vi "WriteSettings.vi"(8 "error in (no error)":errorcluster, 10 "Settings":T1, 11 "Controller in":refnum<class "Controller.lvclass">) -> (0 "error out":errorcluster, 3 "Controller out":refnum<class "Controller.lvclass">)   [LabVIEW 2024, in "GUI.lvlib" / "Controller.lvclass"]
uses:
  Controller.lvclass
  Controller.lvclass/Controller.ctl
  <vilib>/drjdpowell/SQLite Library/SQLite.lvlib
  <vilib>/drjdpowell/SQLite Library/SQL Connection/Execute SQL (No results).vi
  <vilib>/drjdpowell/SQLite Library/SQL Connection/Connection.lvclass
  TypeDefs/Settings.ctl
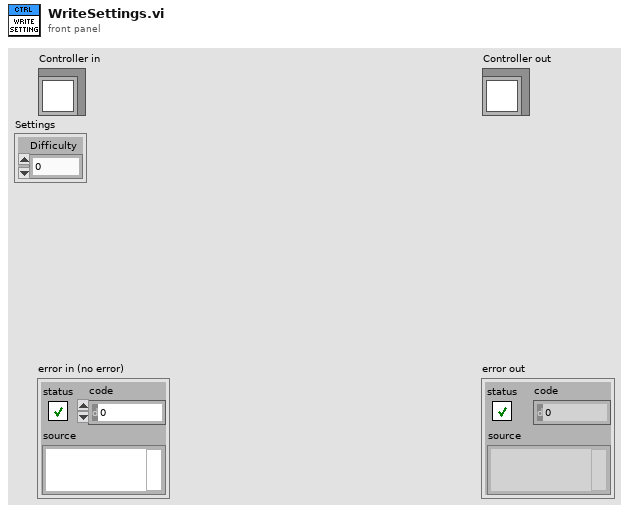
[diagram p1: front panel]
types:
  T1 = typedef "Settings.ctl" = cluster{"Difficulty":i32}
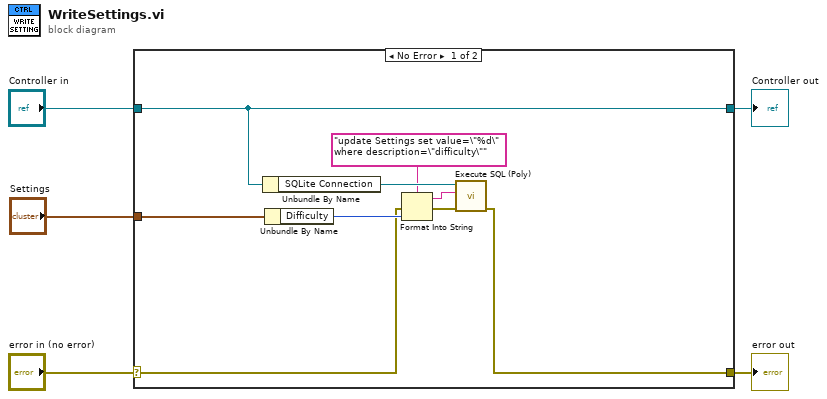
[diagram p0: block diagram]
diagram:
  n1 = case shown="No Error" "error in (no error)" {
    selector: "error in (no error)" -> [w8 w16]
    tunnel: [w7 w16] -> w4
    tunnel: [w14 w15] -> w2
    tunnel: "Controller in" -> [w14 w15]
    tunnel: "Settings" -> [w10 _]
    frame No Error {
      n2 = Unbundle By Name(w14) -> ("SQLite Connection"=w13:refnum<class "Connection.lvclass">)
      n3 = Unbundle By Name(w10) -> ("Difficulty"=w9:i32)
      n4 = Format Into String(format string="update Settings set value=\"%d\" where description=\"difficulty\"", error in=w8, w9) -> (resulting string=w6:string, error out=w11:errorcluster)  [unwired: 1 in]
      n5 = call-poly <vilib>:"Execute SQL (Poly).vi"("error in (no error)"=w11, "SQL"=w6, "SQLite Connection in"=w13) -> ("error out"=w7:errorcluster)  [unwired: 7 in, 1 out]
    }
    frame Error {
    }
  }
  "error out" <- w4
  "Controller out" <- w2
